vi "이벤트 루프 횟수 카운트.vi"() -> ()   [LabVIEW 2016]
panel:
  in  "불리언 3":bool
  in  "불리언 2":bool
  in  "불리언":bool
  out "숫자형":u32
  out "정적 횟수":u8
  out "동적 횟수":u8
  out "유턴 횟수":u8
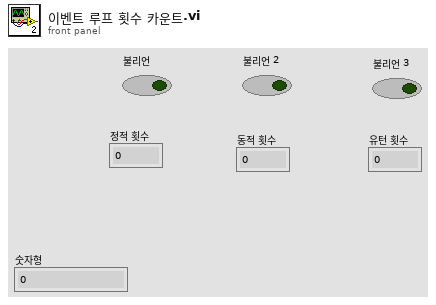
[diagram p1: front panel]
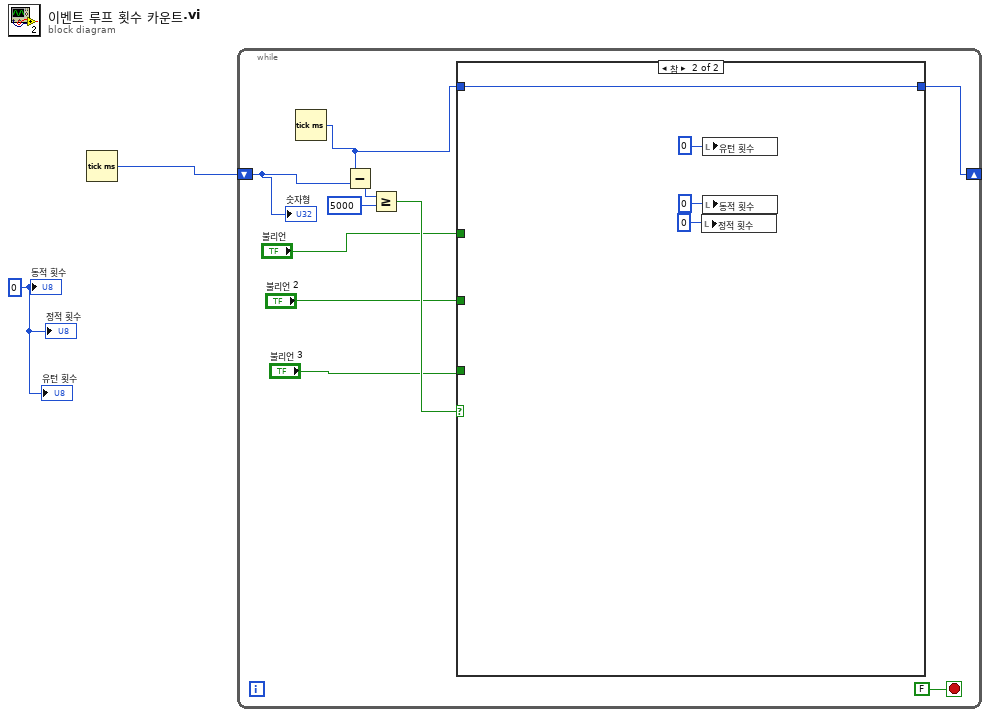
[diagram p0: block diagram]
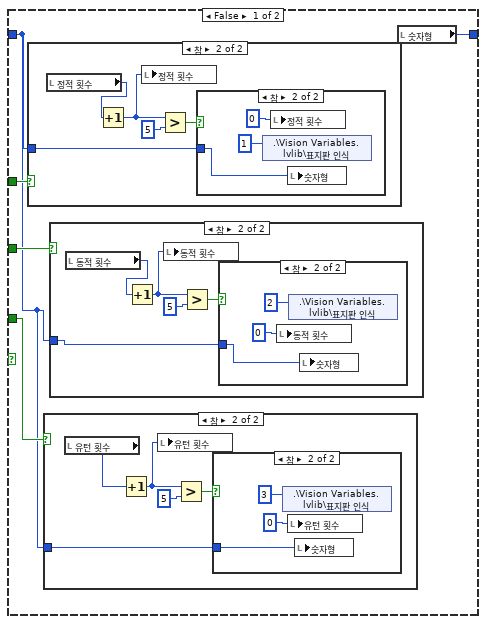
[diagram p2: hidden frame]
diagram:
  w1 = u8 0 ("동적 횟수")
  n1 = Tick Count (ms)() -> (millisecond timer value=w2:u32)
  n2 = while {
    shift-right: [w7] -> _
    shift-left: w2 -> [w6]
    stop <- FALSE stop-if-true
    n3 = Tick Count (ms)() -> (millisecond timer value=w8:u32)
    n4 = Subtract(x=w8, y=w6) -> (x-y=w11:u32)
    n5 = Greater Or Equal?(x=w11, y=u32 5000 ("x-y")) -> (x >= y?=w9:bool)
    n6 = case shown="참" w9 {
      tunnel: "불리언" -> [w17 _]
      tunnel: "불리언 2" -> [w16 _]
      tunnel: "불리언 3" -> [w15 _]
      tunnel: w8 -> [w13 w45]
      tunnel: [w14 w45] -> w7
      frame False {
        n7 = case shown="참" w17 {
          tunnel: w13 -> [_ w34]
          frame False {
          }
          frame True {
            n8 = local read "정적 횟수"() -> (w35:u8)
            n9 = Increment(x=w35) -> (x+1=w37:u8)
            n10 = local write "정적 횟수"(w37) -> ()
            n11 = Greater?(x=w37, y=u8 5) -> (0:w36:bool)
            n12 = case shown="참" w36 {
              tunnel: w34 -> [_ w39]
              frame False {
              }
              frame True {
                n13 = shared-variable ".\\Vision Variables.lvlib\\표지판 인식"(u8 1 ("표지판 인식")) -> ()  [unwired: 1 in, 1 out]
                n14 = local write "정적 횟수"(u8 0 ("정적 횟수")) -> ()
                n15 = local write "숫자형"(w39) -> ()
              }
            }
          }
        }
        n16 = case shown="참" w15 {
          tunnel: w13 -> [_ w18]
          frame False {
          }
          frame True {
            n17 = local read "유턴 횟수"() -> (w19:u8)
            n18 = Increment(x=w19) -> (x+1=w21:u8)
            n19 = local write "유턴 횟수"(w21) -> ()
            n20 = Greater?(x=w21, y=u8 5) -> (0:w20:bool)
            n21 = case shown="참" w20 {
              tunnel: w18 -> [_ w23]
              frame False {
              }
              frame True {
                n22 = shared-variable ".\\Vision Variables.lvlib\\표지판 인식"(u8 3 ("표지판 인식")) -> ()  [unwired: 1 in, 1 out]
                n23 = local write "유턴 횟수"(u8 0 ("정적 횟수")) -> ()
                n24 = local write "숫자형"(w23) -> ()
              }
            }
          }
        }
        n25 = case shown="참" w16 {
          tunnel: w13 -> [_ w26]
          frame False {
          }
          frame True {
            n26 = local read "동적 횟수"() -> (w27:u8)
            n27 = Increment(x=w27) -> (x+1=w29:u8)
            n28 = local write "동적 횟수"(w29) -> ()
            n29 = Greater?(x=w29, y=u8 5) -> (0:w28:bool)
            n30 = case shown="참" w28 {
              tunnel: w26 -> [_ w31]
              frame False {
              }
              frame True {
                n31 = local write "동적 횟수"(u8 0 ("정적 횟수")) -> ()
                n32 = shared-variable ".\\Vision Variables.lvlib\\표지판 인식"(u8 2 ("표지판 인식")) -> ()  [unwired: 1 in, 1 out]
                n33 = local write "숫자형"(w31) -> ()
              }
            }
          }
        }
        n34 = local read "숫자형"() -> (w14:u32)
      }
      frame True {
        n35 = local write "정적 횟수"(u8 0 ("정적 횟수")) -> ()
        n36 = local write "유턴 횟수"(u8 0 ("정적 횟수")) -> ()
        n37 = local write "동적 횟수"(u8 0 ("정적 횟수")) -> ()
      }
    }
    "숫자형" <- w6
  }
  "동적 횟수" <- w1
  "정적 횟수" <- w1
  "유턴 횟수" <- w1
